vi "Self Queue.vi"(9 "Priority?":bool, 10 "Msg Strategy":refnum<class "Msg Strategy.lvclass">, 11 "Base Queue in":refnum<class "Base Queue.lvclass">) -> (3 "Base Queue out":refnum<class "Base Queue.lvclass">)   [LabVIEW 2021, in "jettl.lvlib" / "Base Queue.lvlib" / "Base Queue.lvclass"]
uses:
  Base Queue.lvclass
  Msg Strategy/Msg Strategy.lvclass
  Base Queue.lvclass/Base Queue.ctl
  Self Queue/Self Queue.lvlib
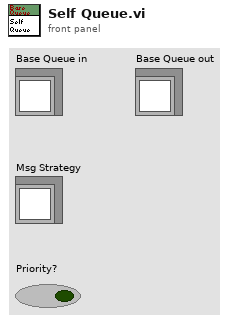
[diagram p1: front panel]
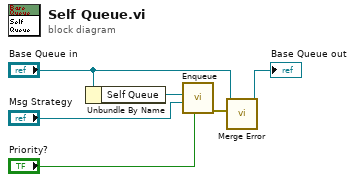
[diagram p0: block diagram]
diagram:
  n1 = Unbundle By Name("Base Queue in") -> ("Self Queue"=w6:refnum<data-value>)
  n2 = call "Enqueue.vi"("Priority?"="Priority?", "Msg Strategy"="Msg Strategy", "Self Queue"=w6) -> ("error out"=w5:errorcluster)  [unwired: 8 in]
  n3 = call-dynamic "Merge Error.vi"("Error"=w5, "Base Queue in"="Base Queue in") -> ("Base Queue out"=→"Base Queue out":refnum<class "Base Queue.lvclass">)  [unwired: 9 in]
